vi "Open first FITS Reference.vi"(8 "error in (no error)":errorcluster, 11 "Save Image in":refnum<class "Save Image.lvclass">) -> (0 "error out":errorcluster, 3 "Save Image out":refnum<class "Save Image.lvclass">)   [LabVIEW 2018, in "Save Image.lvclass"]
uses:
  Save Image.lvclass
  <userlib>/gfitsio/gfitsio.lvlib
  Simulated_Header/Simulated_Header.lvclass
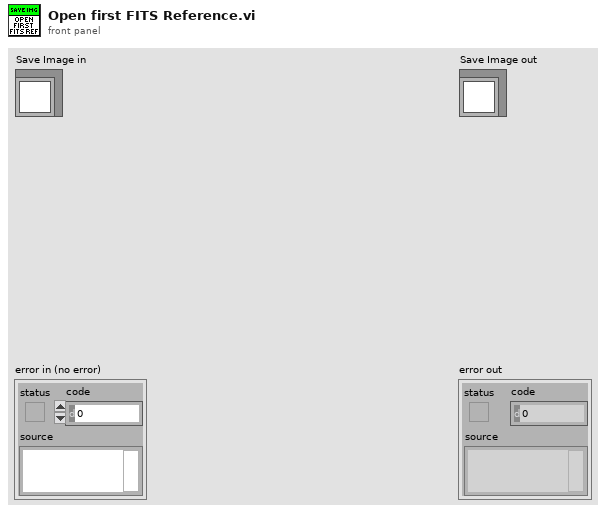
[diagram p1: front panel]
types:
  T1 = enum16{"open", "open or create", "create or replace", "create", "open (read only)"}
  T2 = typedef "gfitsio.lvlib/gfitsio-refnum.ctl" = refnum<k1>
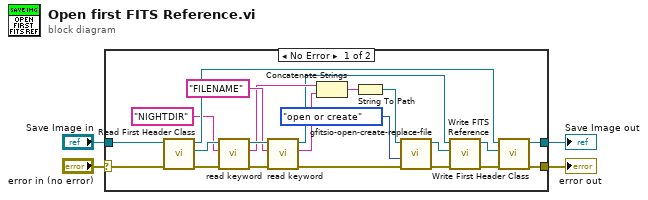
[diagram p0: block diagram]
diagram:
  n1 = case shown="No Error" "error in (no error)" {
    selector: "error in (no error)" -> [w17 w28]
    tunnel: [w20 w28] -> w3
    tunnel: [w21 w27] -> w1
    tunnel: "Save Image in" -> [w25 w27]
    frame No Error {
      n2 = call "Read First Header Class.vi"("error in (no error)"=w17, "Save Image in"=w25) -> ("error out"=w14:errorcluster, "Simulated_Header.lvclass"=w10:refnum<class "Simulated_Header.lvclass">, "Save Image out"=w22:refnum<class "Save Image.lvclass">)  [unwired: 7 in]
      n3 = call "read keyword.vi"("error in (no error)"=w14, "keyword"="NIGHTDIR", "Simulated_Header in"=w10) -> ("error out"=w13:errorcluster, "value"=w7:string, "Simulated_Header out"=w11:refnum<class "Simulated_Header.lvclass">)  [unwired: 6 in]
      n4 = call "read keyword.vi"("error in (no error)"=w13, "keyword"="FILENAME", "Simulated_Header in"=w11) -> ("error out"=w12:errorcluster, "value"=w6:string, "Simulated_Header out"=w5:refnum<class "Simulated_Header.lvclass">)  [unwired: 6 in]
      n5 = Concatenate Strings(w7, w6) -> (w16:string)
      n6 = String To Path(string=w16) -> (path=w15:path)
      n7 = call <userlib>:"gfitsio-open-create-replace-file.vi"("error in (no error)"=w12, "function (open)"=T1."open or create", "file path (dialog if empty)"=w15) -> ("error out"=w23:errorcluster, "gfits refnum"=w24:T2)  [unwired: 6 in, 1 out]
      n8 = call "Write FITS Reference.vi"("error in (no error)"=w23, "gfits refnum"=w24, "Simulated_Header in"=w5) -> ("error out"=w19:errorcluster, "Simulated_Header out"=w18:refnum<class "Simulated_Header.lvclass">)  [unwired: 7 in]
      n9 = call "Write First Header Class.vi"("error in (no error)"=w19, "Simulated_Header.lvclass"=w18, "Save Image in"=w22) -> ("error out"=w20:errorcluster, "Save Image out"=w21:refnum<class "Save Image.lvclass">)  [unwired: 7 in]
    }
    frame Error {
    }
  }
  "error out" <- w3
  "Save Image out" <- w1
